vi "Import - Tx Packets.vi"(7 "Tx Packets":T1 {"Tx Packet Data"."Endianness" items=["big-endian"=0, "little-endian"=2]}, 8 "error in (no error)":errorcluster, 11 "Device Item Ref in":T11 format="%.0x") -> (0 "error out":errorcluster)   [LabVIEW 2016, in "UDP-Custom-Device System Explorer.lvlib"]
uses:
  UDP-Custom-Device System Explorer.lvlib
  <vilib>/NI Veristand/Custom Device API/Custom Device Item Ref.ctl
  Types/XML - New/ImpExp - Tx Packets Data.ctl
  <vilib>/NI Veristand/Custom Device API/Custom Device Item Info.ctl
  Types/XML - New/ImpExp - Tx Packet Data.ctl
  Shared/Types/Shared - Channel Data Type.ctl
  Shared/Types/Shared - Buffered.PacketInfo.ctl
  Shared/Types/Shared - Pointer Encoding.ctl
  Shared/Types/Shared - Receive Buffer Options.ctl
  Shared/Types/Shared - Transmit Buffer Options.ctl
  Shared/Types/Shared - Transmit Flag Options.ctl
  Shared/Types/Shared - Transmit Echo Options.ctl
  Property Accessors/Shared Section Accessors.lvlib
  <vilib>/NI VeriStand/Custom Device API/Custom Device API.lvlib
  Shared/UDP-Custom-Device Shared.lvlib
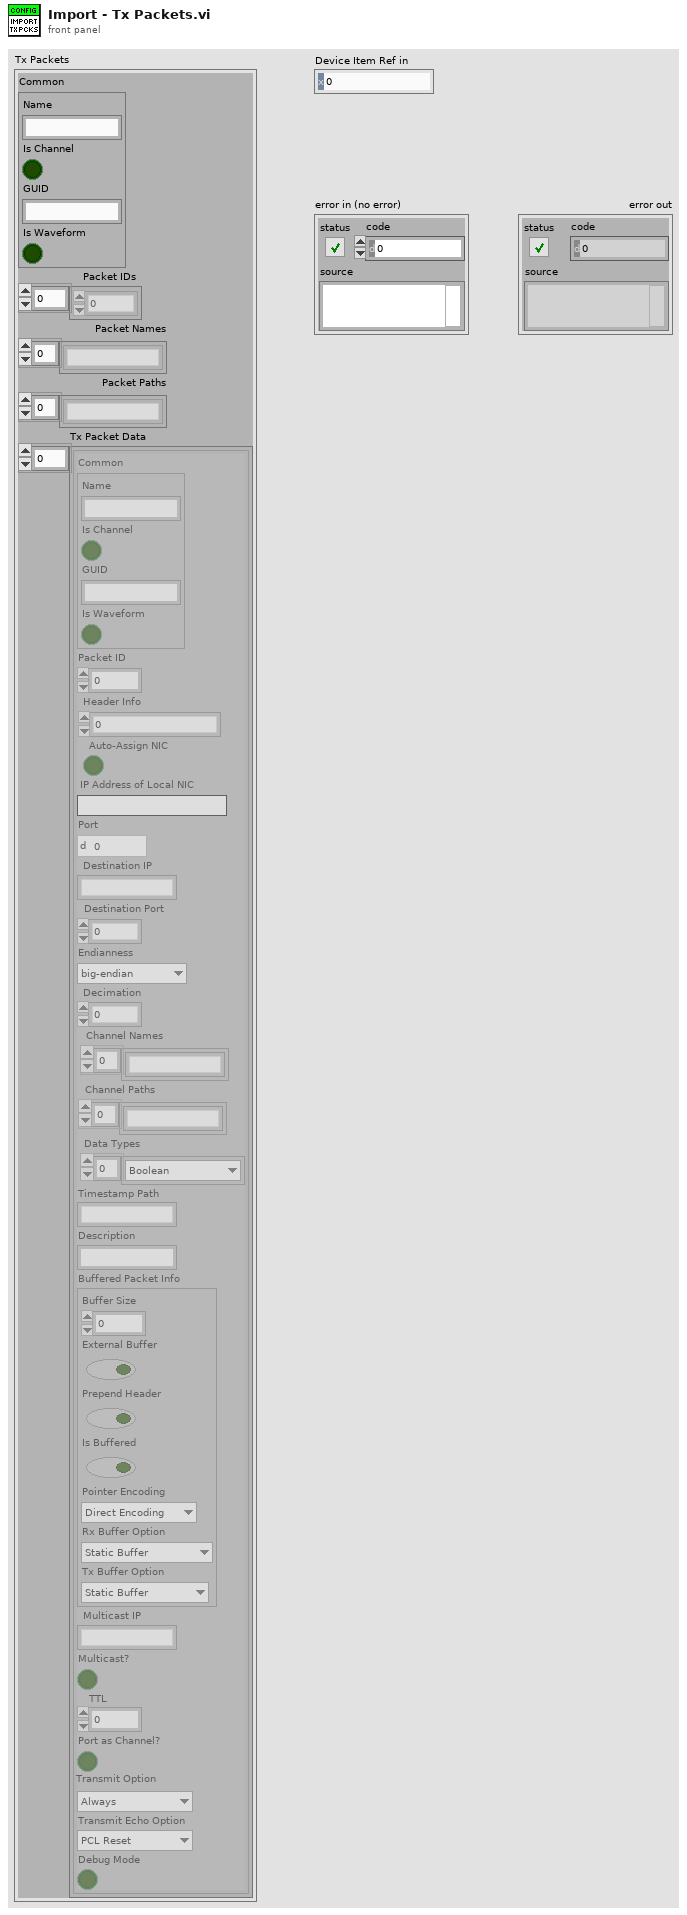
[diagram p1: front panel]
types:
  T1 = typedef "UDP-Custom-Device System Explorer.lvlib/ImpExp - Tx Packets Data.ctl" = cluster{"Common":T2, "Packet IDs":i32[], "Packet Names":string[], "Packet Paths":string[], "Tx Packet Data":T3[]}
  T2 = typedef "Custom Device API.lvlib/Custom Device Item Info.ctl" = cluster{"Name":string, "Is Channel":bool, "GUID":string, "Is Waveform":bool}
  T3 = typedef "UDP-Custom-Device System Explorer.lvlib/ImpExp - Tx Packet Data.ctl" = cluster{"Common":T2, "Packet ID":i32, "Header Info":u32, "Auto-Assign NIC":bool, "IP Address of Local NIC":string, "Port":u16, "Destination IP":string, "Destination Port":u16, "Endianness":u16, "Decimation":u16, "Channel Names":string[], "Channel Paths":string[], "Data Types":T4[], "Timestamp Path":string, "Description":string, "Buffered Packet Info":T5, "Multicast IP":string, "Multicast?":bool, "TTL":u16, "Port as Channel?":bool, "Transmit Option":T9, "Transmit Echo Option":T10, "Debug Mode":bool}
  T4 = typedef "UDP-Custom-Device Shared.lvlib/Shared - Channel Data Type.ctl" = enum16{"Boolean", "Single", "Double", "I8", "I16", "I32", "I64", "U8", "U16", "U32", "U64"}
  T5 = typedef "UDP-Custom-Device Shared.lvlib/Shared - Buffered.PacketInfo.ctl" = cluster{"Buffer Size":i32, "External Buffer":bool, "Prepend Header":bool, "Is Buffered":bool, "Pointer Encoding":T6, "Rx Buffer Option":T7, "Tx Buffer Option":T8}
  T6 = typedef "UDP-Custom-Device Shared.lvlib/Shared - Pointer Encoding.ctl" = enum16{"Direct Encoding", "Conversion Encoding"}
  T7 = typedef "UDP-Custom-Device Shared.lvlib/Shared - Receive Buffer Options.ctl" = enum16{"Static Buffer", "Circular Buffer", "Circular Buffer + Size"}
  T8 = typedef "UDP-Custom-Device Shared.lvlib/Shared - Transmit Buffer Options.ctl" = enum16{"Static Buffer", "FIFO Buffer", "FIFO Buffer + Port"}
  T9 = typedef "UDP-Custom-Device Shared.lvlib/Shared - Transmit Flag Options.ctl" = enum16{"Always", "One-Shot", "Toggle"}
  T10 = typedef "UDP-Custom-Device Shared.lvlib/Shared - Transmit Echo Options.ctl" = enum16{"PCL Reset", "Counter", "Mirror"}
  T11 = typedef "Custom Device API.lvlib/Custom Device Item Ref.ctl" = u64
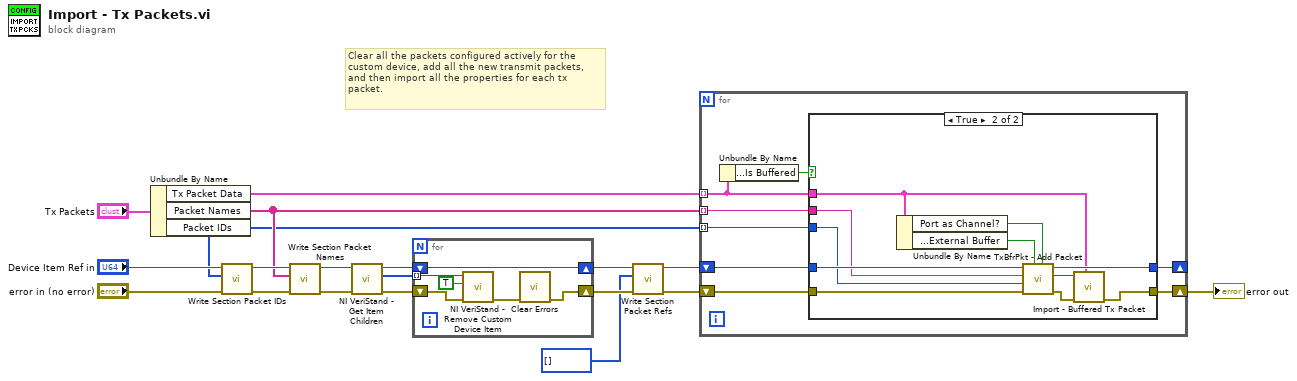
[diagram p0: block diagram]
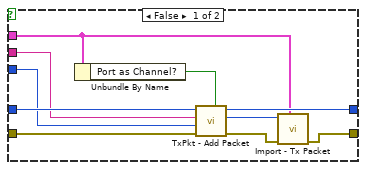
[diagram p2: hidden frame]
diagram:
  # "Clear all the packets configured actively for the\ncustom device, add all the new transmit packets,\nand then import all the properties for each tx\npacket."
  n1 = Unbundle By Name("Tx Packets") -> ("Tx Packet Data"=w14:T3[], "Packet Names"=w8:string[], "Packet IDs"=w7:i32[])
  n2 = call "Write Section Packet IDs.vi"("error in (no error)"="error in (no error)", "Packet IDs"=w7, "Node Ptr"="Device Item Ref in") -> ("error out"=w15:errorcluster, "Node Ptr out"=w16:T11)  [unwired: 7 in]
  n3 = call "Write Section Packet Names.vi"("error in (no error)"=w15, "Packet Names"=w8, "Node Ptr"=w16) -> ("error out"=w12:errorcluster, "Node Ptr out"=w13:T11)  [unwired: 7 in]
  n4 = call <vilib>:"NI VeriStand - Get Item Children.vi"("error in (no error)"=w12, "Item Ref in"=w13) -> ("error out"=w11:errorcluster, "Child Refs"=w10:T11[], "Item Ref out"=w9:T11)  [unwired: 6 in, 1 out]
  n5 = for {
    shift-right: [w20] -> w3
    shift-left: w11 -> [w25]
    tunnel: w10 -> [w24] mode=indexing
    shift-right: [w23] -> w5
    shift-left: w9 -> [w23]
    n6 = call <vilib>:"NI VeriStand - Remove Custom Device Item.vi"("error in (no error)"=w25, "Force Delete (F)"=TRUE, "Item Ref in"=w24) -> ("error out"=w21:errorcluster)  [unwired: 7 in, 1 out]
    n7 = call <vilib>:"Clear Errors.vi"("error in (no error)"=w21) -> ("error out"=w20:errorcluster)  [unwired: 5 in, 1 out]
  }
  n8 = call "Write Section Packet Refs.vi"("error in (no error)"=w3, "Dependent Node Refs"=T11[] [], "Node Ptr"=w5) -> ("error out"=w2:errorcluster, "Node Ptr out"=w4:T11)  [unwired: 7 in]
  n9 = for {
    shift-right: [w29] -> _
    shift-left: w4 -> [w33]
    shift-right: [w28] -> w6
    shift-left: w2 -> [w32]
    tunnel: w14 -> [w27] mode=indexing
    tunnel: w8 -> [w31] mode=indexing
    tunnel: w7 -> [w30] mode=indexing
    n10 = Unbundle By Name(w27) -> ("Buffered Packet Info.Is Buffered"=w26:bool)
    n11 = case shown="True" w26 {
      tunnel: w33 -> [w43 w54]
      tunnel: w32 -> [w42 w53]
      tunnel: w31 -> [w41 w52]
      tunnel: w30 -> [w40 w51]
      tunnel: [w39 w47] -> w29
      tunnel: [w36 w48] -> w28
      tunnel: w27 -> [w35 w46]
      frame False {
        n12 = Unbundle By Name(w35) -> ("Port as Channel?"=w34:bool)
        n13 = call "TxPkt - Add Packet.vi"("Add Port Channel"=w34, "error in (no error)"=w42, "New Packet ID"=w40, "New Packet Name"=w41, "Item Ref in"=w43) -> ("error out"=w37:errorcluster, "New Packet Ref"=w38:T11, "Item Ref Out"=w39:T11)  [unwired: 4 in]
        n14 = call "Import - Tx Packet.vi"("Tx Packet"=w35, "error in (no error)"=w37, "Device Item Ref in"=w38) -> ("error out"=w36:errorcluster)  [unwired: 8 in]
      }
      frame True {
        n15 = Unbundle By Name(w46) -> ("Port as Channel?"=w44:bool, "Buffered Packet Info.External Buffer"=w45:bool)
        n16 = call "TxBfrPkt - Add Packet.vi"("Add Port Channel?"=w44, "Ext Buffer?"=w45, "error in (no error)"=w53, "New Packet ID"=w51, "New Packet Name"=w52, "Item Ref in"=w54) -> ("error out"=w49:errorcluster, "New Packet Ref"=w50:T11, "Item Ref Out"=w47:T11)  [unwired: 3 in]
        n17 = call "Import - Buffered Tx Packet.vi"("Tx Packet"=w46, "error in (no error)"=w49, "Device Item Ref in"=w50) -> ("error out"=w48:errorcluster)  [unwired: 8 in]
      }
    }
  }
  "error out" <- w6
